vi "Synchronize Control VI.vi"(8 "error in (no error)":errorcluster, 10 "Control Destination":path, 11 "Control in":refnum<class "Control.lvclass">) -> (0 "error out":errorcluster, 3 "Control out":refnum<class "Control.lvclass">)   [LabVIEW 2013, in "Control.lvclass"]
doc: "Creates the customized button on disk and/or on front panel."
uses:
  Control.lvclass
  <vilib>/Utility/miscctls.llb/LVFontTypeDef.ctl
  <vilib>/Utility/miscctls.llb/LVPositionTypeDef.ctl
  <userlib>/BitMan/BitMap class/BitMap.lvclass
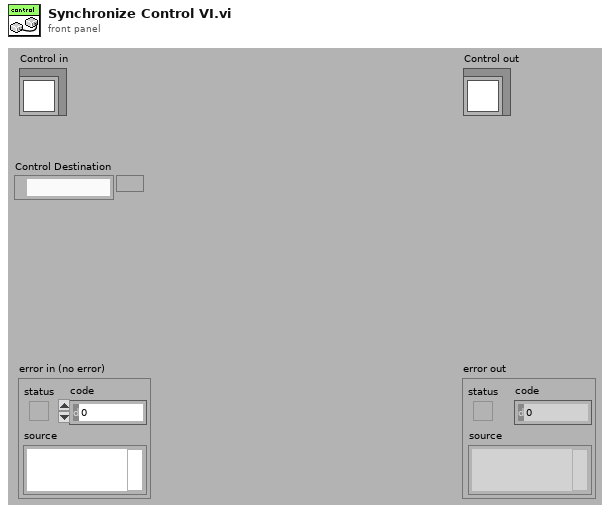
[diagram p1: front panel]
types:
  T1 = typedef "LVFontTypeDef.ctl" = cluster{"Font Name":string, "Size":u16, "Bold":bool, "Italic":bool, "Underline":bool, "Strikeout":bool, "Color":u32}
  T2 = typedef "LVPositionTypeDef.ctl" = cluster{"Left":i32, "Top":i32}
  T3 = typedef "imagedata.ctl" = cluster{"image type":i32, "image depth":i32, "image":u8[], "mask":u8[], "colors":u32[], "Rectangle":cluster{"left":i16, "top":i16, "right":i16, "bottom":i16}}
  T4 = typedef "Control.lvclass/BX.Orientation__LCR _Modified.ctl" = u8
  T5 = cluster{"left":i16, "top":i16, "right":i16, "bottom":i16}
  T6 = typedef "Control.lvclass/_ui_tools_font.ctl" = cluster{"Font Name:":string, "Size":i16, "Strikeout?":bool, "Italic?":bool, "Underline?":bool, "Outline?":bool, "Shadow?":bool, "Bold?":bool}
  T7 = typedef "Control.lvclass/TypeDef_Action.ctl" = u16
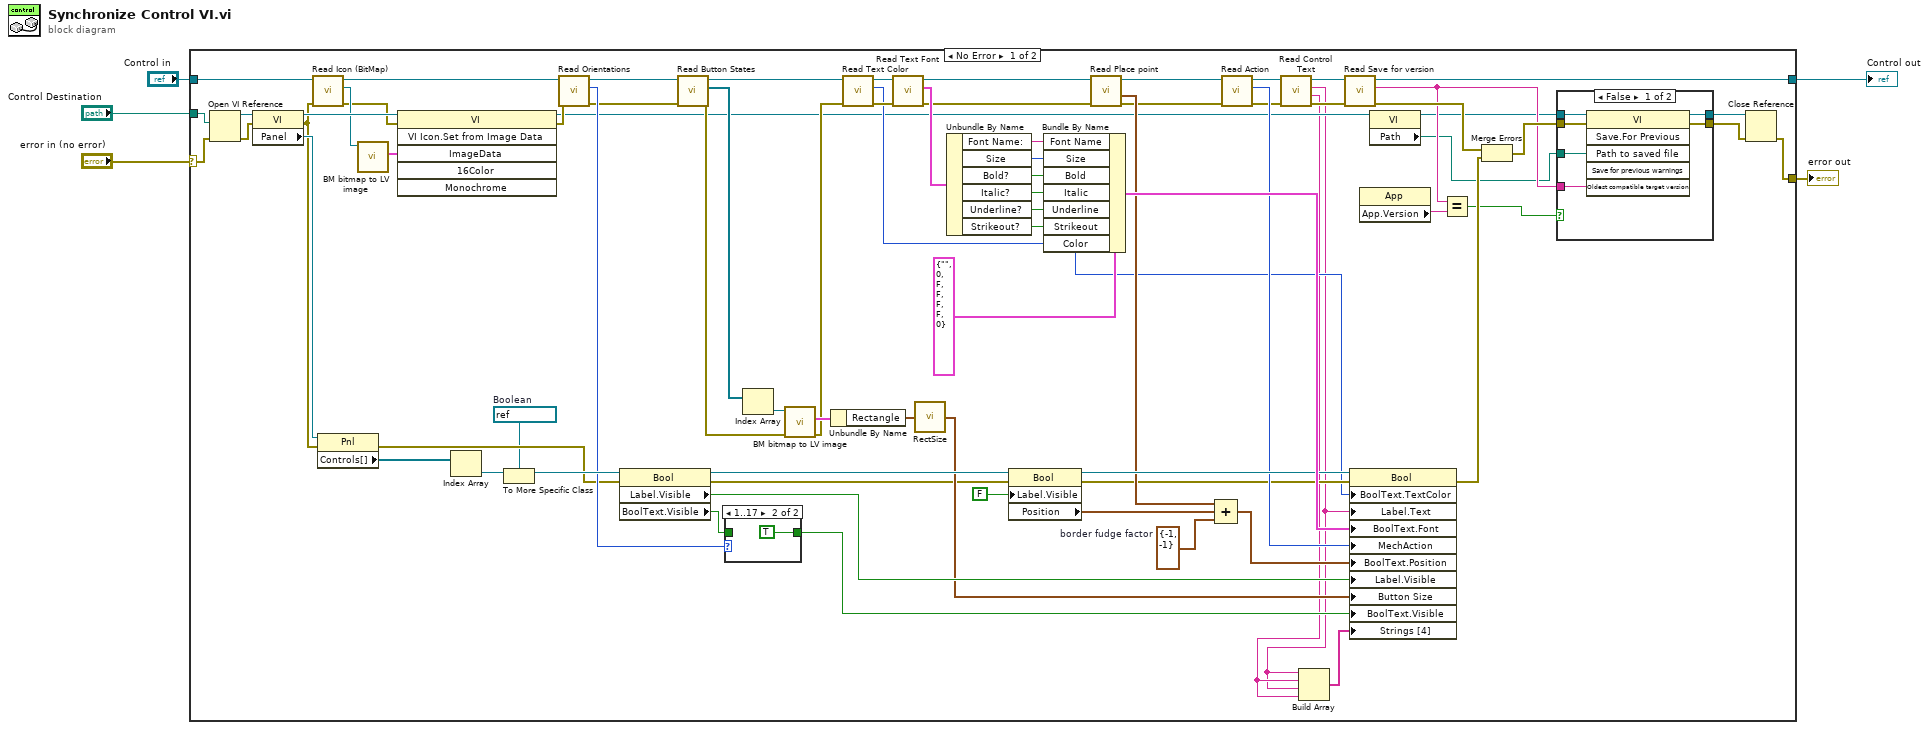
[diagram p0: block diagram]
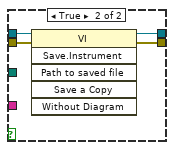
[diagram p2: hidden frame]
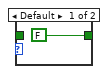
[diagram p3: hidden frame]
diagram:
  n1 = case shown="No Error" "error in (no error)" {
    selector: "error in (no error)" -> [w75 w97]
    tunnel: [w76 w97] -> w4
    tunnel: [w18 w96] -> w2
    tunnel: "Control in" -> [w49 w96]
    tunnel: "Control Destination" -> [w78 _]
    frame No Error {
      w8 = refnum<vi> refnum  # Boolean
      w20 = T2 {"Left"=-1, "Top"=-1}  # border fudge factor
      n2 = Open VI Reference(vi path=w78, error in (no error)=w75) -> (vi reference=w83:refnum<vi>, error out=w74:errorcluster)  [unwired: 4 out]
      n3 = property class="VI"(reference=w83, error in=w74) -> (reference out=w62:refnum<vi>, error out=w33:errorcluster, "Panel"=w82:refnum<vi>)
      n4 = call-dynamic "Read Icon (BitMap).vi"("error in (no error)"=w33, "Control in"=w49) -> ("error out"=w38:errorcluster, "Icon (BitMap) False"=w47:refnum<class "BitMap.lvclass">, "Control out"=w48:refnum<class "Control.lvclass">)  [unwired: 7 out]
      n5 = property class="Pnl"(reference=w82, error in=w33) -> (error out=w32:errorcluster, "Controls[]"=w81:refnum<vi>[])  [unwired: 1 out]
      n6 = call <userlib>:"BM bitmap to LV image.vi"("BitMap in"=w47) -> ("LV image data"=w63:T3)  [unwired: 2 in, 8 out]
      n7 = invoke class="VI" method="VI Icon.Set from Image Data"(reference=w62, error in=w38, "ImageData"=w63) -> (reference out=w12:refnum<vi>, error out=w37:errorcluster)  [unwired: 3 in, 4 out]
      n8 = Index Array(array=w81) -> (element=w80:refnum<vi>)  [unwired: 1 in]
      n9 = To More Specific Class(target class=w8, reference=w80) -> (specific class reference=w57:refnum<vi>)  [unwired: 1 in, 1 out]
      n10 = call-dynamic "Read Orientations.vi"("error in (no error)"=w37, "Control in"=w48) -> ("error out"=w36:errorcluster, "Orientations"=w53:T4, "Control out"=w44:refnum<class "Control.lvclass">)  [unwired: 7 out]
      n11 = property class="Bool"(reference=w57, error in=w32) -> (reference out=w56:refnum<vi>, error out=w30:errorcluster, "Label.Visible"=w52:bool, "BoolText.Visible"=w51:bool)
      n12 = call-dynamic "Read Button States.vi"("error in (no error)"=w36, "Control in"=w44) -> ("error out"=w31:errorcluster, "Button States"=w43:refnum<class "BitMap.lvclass">[], "Control out"=w25:refnum<class "Control.lvclass">)  [unwired: 7 out]
      n13 = case shown="1..17" w53 {
        tunnel: [FALSE TRUE] -> w50
        tunnel: w51 -> [_ _]
        frame Default {
        }
        frame 1..17 {
        }
      }
      n14 = Index Array(array=w43) -> (element=w55:refnum<class "BitMap.lvclass">)  [unwired: 1 in]
      n15 = call <userlib>:"BM bitmap to LV image.vi"("error in (no error)"=w31, "BitMap in"=w55) -> ("error out"=w23:errorcluster, "LV image data"=w54:T3)  [unwired: 1 in, 7 out]
      n16 = Unbundle By Name(w54) -> ("Rectangle"=w46:T5)
      n17 = call-dynamic "Read Text Color.vi"("error in (no error)"=w23, "Control.lvclass in"=w25) -> ("error out"=w22:errorcluster, "Text Color"=w21:u32, "Control.lvclass out"=w24:refnum<class "Control.lvclass">)  [unwired: 7 out]
      n18 = call-dynamic "Read Text Font.vi"("error in (no error)"=w22, "Control in"=w24) -> ("error out"=w35:errorcluster, "Font"=w73:T6, "Control out"=w39:refnum<class "Control.lvclass">)  [unwired: 7 out]
      n19 = call <vilib>:"RectSize.vi"("rect"=w46) -> ("point"=w45:cluster{"x":i16, "y":i16})
      n20 = Unbundle By Name(w73) -> ("Font Name:"=w71:string, "Size"=w69:i16, "Bold?"=w68:bool, "Italic?"=w67:bool, "Underline?"=w66:bool, "Strikeout?"=w65:bool)
      n21 = property class="Bool"(reference=w56, error in=w30, "Label.Visible"=FALSE) -> (reference out=w64:refnum<vi>, error out=w29:errorcluster, "Position"=w60:T2)
      n22 = Bundle By Name(cluster=T1 {"Font Name"="", "Size"=0, "Bold"=FALSE, "Italic"=FALSE, "Underline"=FALSE, "Strikeout"=FALSE, "Color"=0} ("Boolean Text.Font"), "Font Name"=w71, "Size"=w69, "Bold"=w68, "Italic"=w67, "Underline"=w66, "Strikeout"=w65, "Color"=w21) -> (w70:T1)
      n23 = call-dynamic "Read Place point.vi"("error in (no error)"=w35, "Control in"=w39) -> ("error out"=w34:errorcluster, "Text Point"=w61:cluster{"x":i32, "y":i32}, "Control out"=w42:refnum<class "Control.lvclass">)  [unwired: 7 out]
      n24 = Compound Arithmetic op=ADD(w61, w60, w20) -> (w58:T2)
      n25 = call-dynamic "Read Action.vi"("error in (no error)"=w34, "Control in"=w42) -> ("error out"=w28:errorcluster, "Action"=w40:T7, "Control out"=w41:refnum<class "Control.lvclass">)  [unwired: 7 out]
      n26 = call-dynamic "Read Control Text.vi"("error in (no error)"=w28, "Control in"=w41) -> ("error out"=w17:errorcluster, "True Text"=w9:string, "Control Text"=w6:string, "Control out"=w19:refnum<class "Control.lvclass">)  [unwired: 6 out]
      n27 = Build Array(w6, w9, w6, w9) -> (w7:string[])
      n28 = call-dynamic "Read Save for version.vi"("error in (no error)"=w17, "Control.lvclass in"=w19) -> ("error out"=w16:errorcluster, "Save for version"=w13:string, "Control.lvclass out"=w18:refnum<class "Control.lvclass">)  [unwired: 7 out]
      n29 = property class="Bool"(reference=w64, error in=w29, "BoolText.TextColor"=w21, "Label.Text"=w6, "BoolText.Font"=w70, "MechAction"=w40, "BoolText.Position"=w58, "Label.Visible"=w52, "Button Size"=w45, "BoolText.Visible"=w50, "Strings [4]"=w7) -> (error out=w27:errorcluster)  [unwired: 1 out]
      n30 = property class="App"() -> ("App.Version"=w15:string)  [unwired: 2 in, 2 out]
      n31 = property class="VI"(reference=w12) -> (reference out=w11:refnum<vi>, "Path"=w10:path)  [unwired: 1 in, 1 out]
      n32 = Equal?(x=w13, y=w15) -> (x = y?=w14:bool)
      n33 = Merge Errors(w16, w27) -> (w26:errorcluster)
      n34 = case shown="False" w14 {
        tunnel: [w88 w93] -> w79
        tunnel: [w86 w92] -> w77
        tunnel: w11 -> [w89 w91]
        tunnel: w26 -> [w85 w90]
        tunnel: w13 -> [w87 _]
        tunnel: w10 -> [w84 _]
        frame False {
          n35 = invoke class="VI" method="Save.For Previous"(reference=w89, error in=w85, "Path to saved file"=w84, "Oldest compatible target version"=w87) -> (reference out=w88:refnum<vi>, error out=w86:errorcluster)  [unwired: 2 in, 4 out]
        }
        frame True {
          n36 = invoke class="VI" method="Save.Instrument"(reference=w91, error in=w90) -> (reference out=w93:refnum<vi>, error out=w92:errorcluster)  [unwired: 4 in, 4 out]
        }
      }
      n37 = Close Reference(reference=w79, error in (no error)=w77) -> (error out=w76:errorcluster)
    }
    frame Error {
    }
  }
  "error out" <- w4
  "Control out" <- w2
